vi "VI Tree.vi"   [LabVIEW 2020, in "Agilent 34401.lvlib"]
doc: "This is the instrument driver for the Keysight/Agilent 34401A, 34410A, 34411A, L4411A digital multimeters."
uses:
  Agilent 34401.lvlib
  Data/Read (Math).vi
  Configure/Configure Temperature (RTD).vi
  Data/Read (Transient).vi
  Data/Read (Multiple Points).vi
  Data/Read (Single Point).vi
panel:
  # "(c) 2005-2015 National Instruments.  ALL RIGHTS RESERVED."
  # "SEE DIAGRAM\nFOR VI Tree"
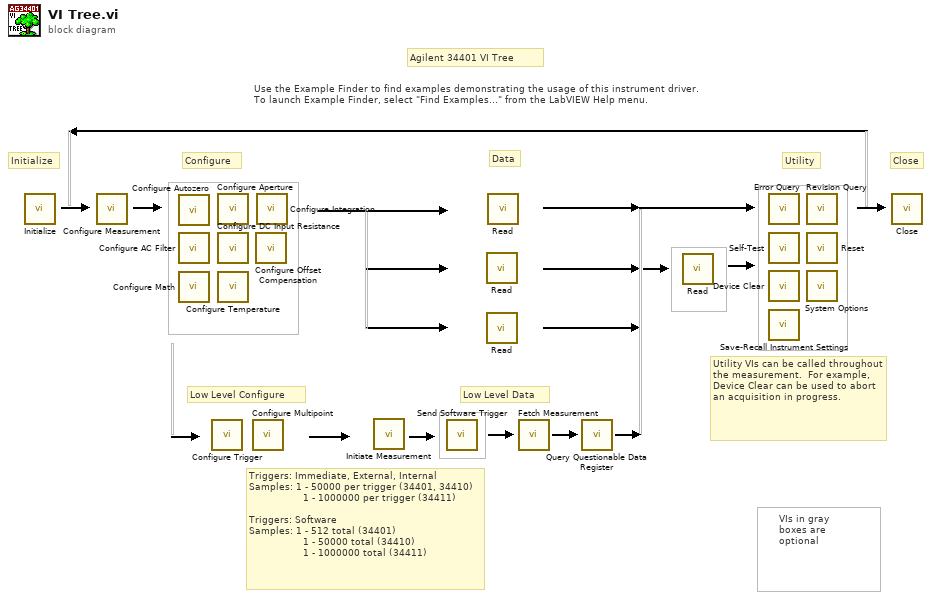
[diagram p0: block diagram]
diagram:
  # "Utility VIs can be called throughout the measurement.  For example, Device Clear can be used to abort an acquisition in progress."
  # "Use the Example Finder to find examples demonstrating the usage of this instrument driver.\nTo launch Example Finder, select \"Find Examples...\" from the LabVIEW Help menu."
  # "Triggers: Immediate, External, Internal\nSamples: 1 - 50000 per trigger (34401, 34410)\n                  1 - 1000000 per trigger (34411)\n\nTriggers: Software\nSamples: 1 - 512 total (34401)\n                  1 - 50000 total (34410)\n                  1 - 1000000 total (34411)"
  # "VIs in gray\nboxes are\noptional"
  # "Agilent 34401 VI Tree"
  # "Low Level Configure"
  # "Low Level Data"
  # "Configure"
  # "Utility"
  # "Data"
  # "Close"
  # "Initialize"
  n1 = call "Initialize.vi"() -> ()  [unwired: 10 in, 2 out]
  n2 = call "Configure Measurement.vi"() -> ()  [unwired: 10 in, 2 out]
  n3 = call "Configure Autozero.vi"() -> ()  [unwired: 10 in, 2 out]
  n4 = call "Configure AC Filter.vi"() -> ()  [unwired: 10 in, 2 out]
  n5 = call "Configure Math.vi"() -> ()  [unwired: 14 in, 2 out]
  n6 = call "Configure Trigger.vi"() -> ()  [unwired: 10 in, 2 out]
  n7 = call "Configure Aperture.vi"() -> ()  [unwired: 10 in, 2 out]
  n8 = call "Configure DC Input Resistance.vi"() -> ()  [unwired: 10 in, 2 out]
  n9 = call-poly "Configure Temperature.vi"() -> ()  [unwired: 14 in, 2 out]
  n10 = call "Configure Multipoint.vi"() -> ()  [unwired: 10 in, 2 out]
  n11 = call "Configure Offset Compensation.vi"() -> ()  [unwired: 10 in, 2 out]
  n12 = call "Configure Integration.vi"() -> ()  [unwired: 10 in, 2 out]
  n13 = call "Initiate Measurement.vi"() -> ()  [unwired: 10 in, 2 out]
  n14 = call "Send Software Trigger.vi"() -> ()  [unwired: 10 in, 2 out]
  n15 = call-poly "Read.vi"() -> ()  [unwired: 9 in, 3 out]
  n16 = call-poly "Read.vi"() -> ()  [unwired: 6 in, 6 out]
  n17 = call-poly "Read.vi"() -> ()  [unwired: 9 in, 3 out]
  n18 = call "Fetch Measurement.vi"() -> ()  [unwired: 8 in, 4 out]
  n19 = call "Query Questionable Data Register.vi"() -> ()  [unwired: 9 in, 3 out]
  n20 = call-poly "Read.vi"() -> ()  [unwired: 4 in, 8 out]
  n21 = call "Error Query.vi"() -> ()  [unwired: 8 in, 4 out]
  n22 = call "Self-Test.vi"() -> ()  [unwired: 8 in, 4 out]
  n23 = call "Device Clear.vi"() -> ()  [unwired: 10 in, 2 out]
  n24 = call "Save-Recall Instrument Settings.vi"() -> ()  [unwired: 10 in, 2 out]
  n25 = call "Revision Query.vi"() -> ()  [unwired: 8 in, 4 out]
  n26 = call "Reset.vi"() -> ()  [unwired: 10 in, 2 out]
  n27 = call "System Options.vi"() -> ()  [unwired: 10 in, 2 out]
  n28 = call "Close.vi"() -> ()  [unwired: 11 in, 1 out]
